vi "H5Topen.vi"(9 "error in (no error)":errorcluster) -> (0 "datatype_id":i32, 6 "error out":errorcluster)   [LabVIEW 2009]
uses:
  hdf5dll.dll
panel:
  in  "tapl_id":i32
  in  "name":string
  in  "loc_id":i32
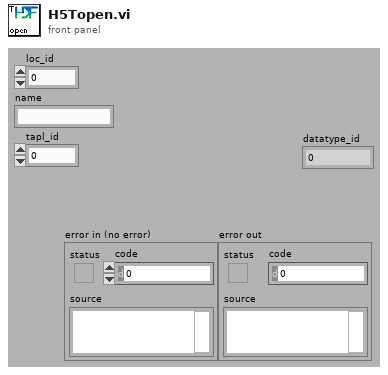
[diagram p1: front panel]
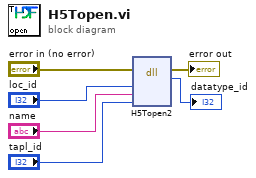
[diagram p0: block diagram]
diagram:
  n1 = dll-call lib="hdf5dll.dll" fn="H5Topen2"(error in="error in (no error)", "loc_id"="loc_id", "name"="name", "tapl_id"="tapl_id") -> (error out=→"error out":errorcluster, "return type"=→"datatype_id":i32)  [unwired: 5 in, 1 out]
